vi "Add Single Event - Slave.vi"(8 "error in (no error)":errorcluster, 10 "Event":T1, 11 "Controller in":refnum<class "Controller.lvclass">) -> (0 "error out":errorcluster, 3 "Controller out":refnum<class "Controller.lvclass">)   [LabVIEW 2019, in "Controller.lvlib" / "Controller.lvclass"]
uses:
  Controller.lvclass
  Sensors/Detector/Event.ctl
  Controller.lvclass/Controller.ctl
  Sensors/Detector/Muon Detector.lvclass
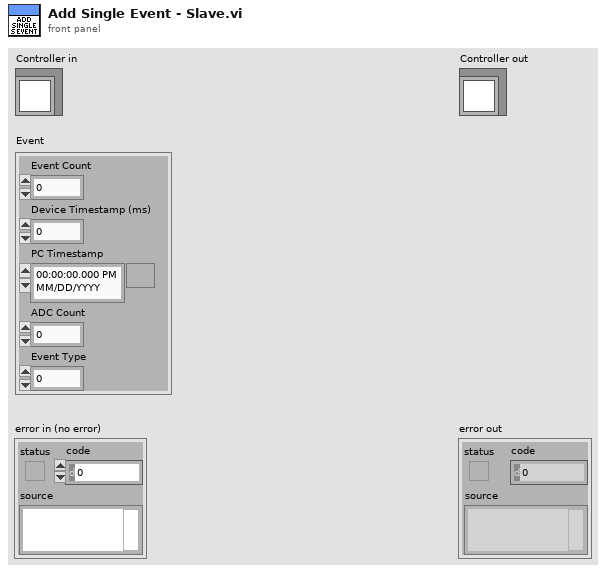
[diagram p1: front panel]
types:
  T1 = typedef "Muon Detector.lvclass/Event.ctl" = cluster{"Event Count":i32, "Device Timestamp (ms)":i32, "PC Timestamp":timestamp, "ADC Count":i32, "Event Type":u8}
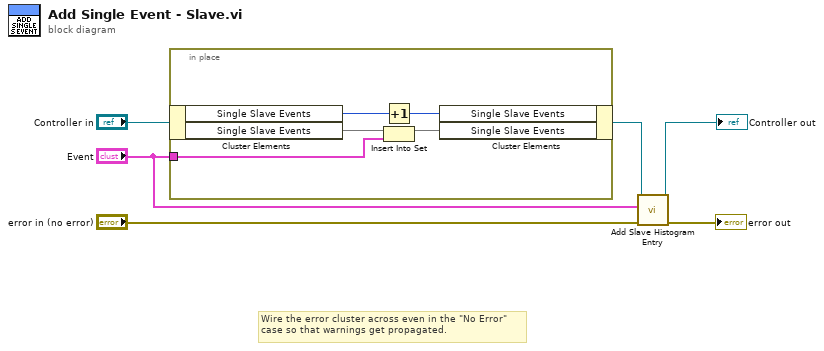
[diagram p0: block diagram]
diagram:
  # "Wire the error cluster across even in the \"No Error\"\ncase so that warnings get propagated."
  n1 = in-place {
    in-place-border: "Event" -> [w10]
    n2 = in-place-cluster #1("Controller in") -> ("Single Slave Events"=w8:i32, "Single Slave Events"=w11:set{T1})
    n3 = Increment(x=w8) -> (x+1=w7:i32)
    n4 = Insert Into Set(10:w10, 11:w11) -> (3:w9:set{T1})  [unwired: 1 out]
    n5 = in-place-cluster #1("Single Slave Events"=w7, "Single Slave Events"=w9) -> (w3:refnum<class "Controller.lvclass">)
  }
  n6 = call "Add Slave Histogram Entry.vi"("error in (no error)"="error in (no error)", "Event"="Event", "Controller in"=w3) -> ("error out"=→"error out":errorcluster, "Controller out"=→"Controller out":refnum<class "Controller.lvclass">)  [unwired: 7 in]
